vi "SolenoidSet_Double.vi"(1 "Solenoid 2":string, 2 "Solenoid 1":string, 3 "Switch To":bool) -> ()   [LabVIEW 2016]
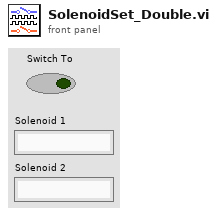
[diagram p1: front panel]
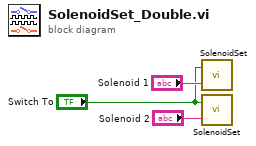
[diagram p0: block diagram]
diagram:
  n1 = call "SolenoidSet.vi"("String"="Solenoid 1", "Boolean"="Switch To") -> ()
  n2 = call "SolenoidSet.vi"("String"="Solenoid 2", "Boolean"="Switch To") -> ()
